vi "Find Type.vi"(8 "error in":errorcluster, 11 "Actor In":refnum<class "Actor.lvclass">) -> (0 "error out":errorcluster, 1 "Type Found?":bool, 2 "Entity Type":T1, 3 "Actor Out":refnum<class "Actor.lvclass">)   [LabVIEW 2020]
doc: "Determines the type of <b>Actor In</b>"
uses:
  <vilib>/ActorFramework/Actor/Actor.lvclass
  Classes/Coffee Shop/Entity Types.ctl
  Classes/Person/Person.lvclass
  Classes/Customer/Customer.lvclass
  Classes/Worker/Worker.lvclass
  Classes/Worker/Barista/Barista.lvclass
  Classes/Worker/Cashier/Cashier.lvclass
  Classes/Coffee Shop/Coffee Shop.lvclass
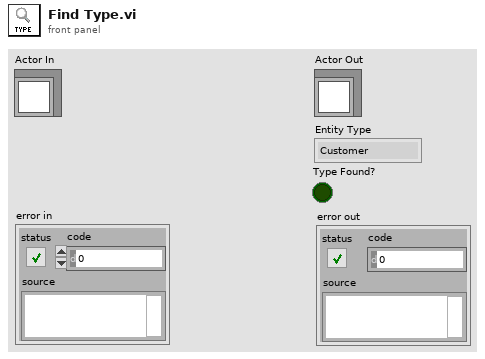
[diagram p1: front panel]
types:
  T1 = typedef "Coffee Shop.lvlib/Coffee Shop.lvclass/Entity Types.ctl" = enum16{"Customer", "Cashier", "Barista"}
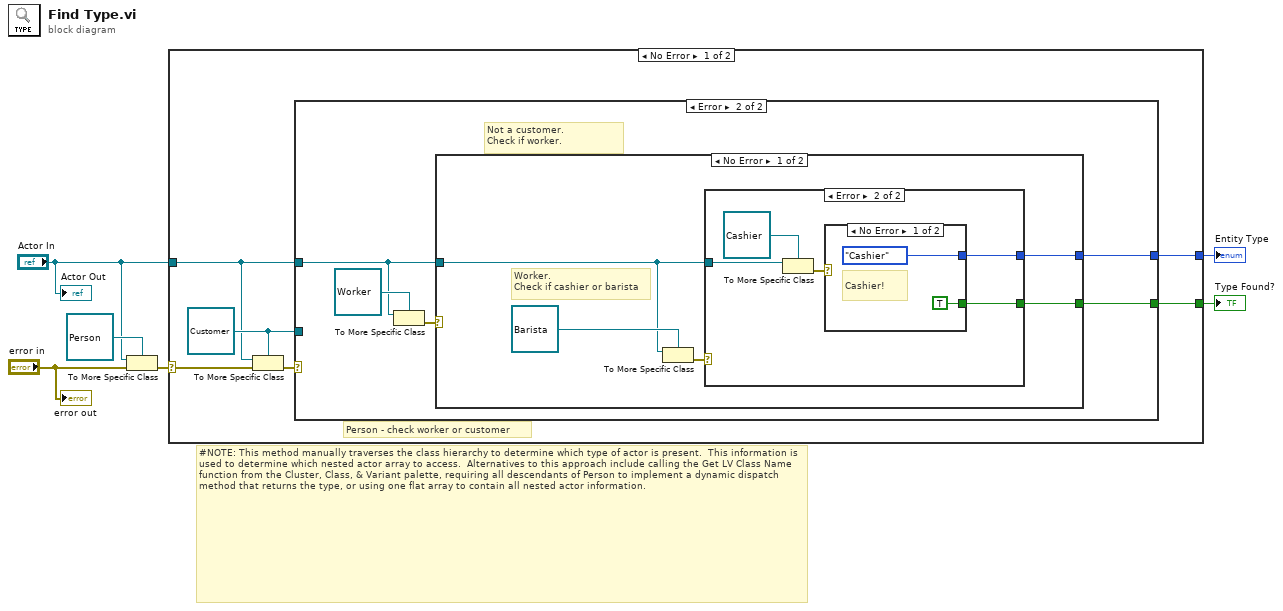
[diagram p0: block diagram]
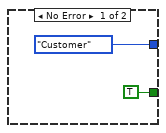
[diagram p2: hidden frame]
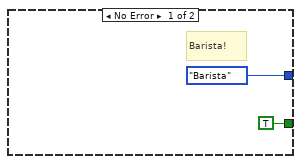
[diagram p3: hidden frame]
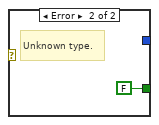
[diagram p4: hidden frame]
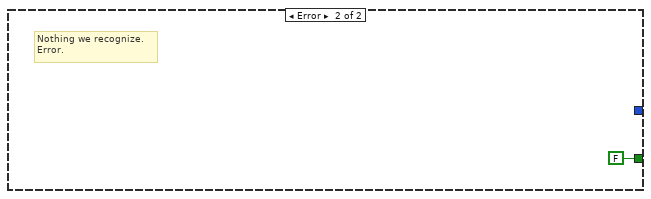
[diagram p5: hidden frame]
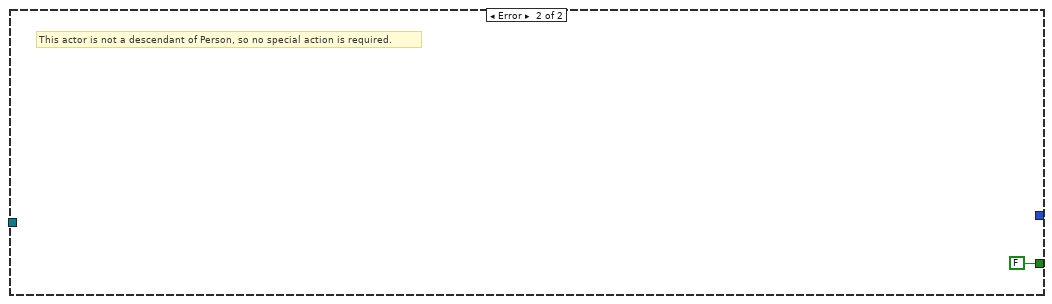
[diagram p6: hidden frame]
diagram:
  # "#NOTE: This method manually traverses the class hierarchy to determine which type of actor is present.  This information is used to determine which nested actor array to access.  Alternatives to this approach include calling the Get LV Class Name function from the Cluster, Class, & Variant palette, requiring all descendants of Person to implement a dynamic dispatch method that returns the type, or using one flat array to contain all nested actor information."
  n1 = To More Specific Class(target class=refnum<class "Person.lvclass"> refnum ("Person.lvclass"), reference="Actor In", error in="error in") -> (error out=w5:errorcluster)  [unwired: 1 out]
  n2 = case shown="No Error" w5 {
    selector: w5 -> [w12 _]
    tunnel: "Actor In" -> [w9 _]
    tunnel: [w8 _] -> w2
    tunnel: [w7 FALSE] -> w3
    frame No Error {
      w10 = refnum<class "Customer.lvclass"> refnum ("Customer.lvlib:Customer.lvclass")
      # "Person - check worker or customer"
      n3 = To More Specific Class(target class=w10, reference=w9, error in=w12) -> (error out=w11:errorcluster)  [unwired: 1 out]
      n4 = case shown="Error" w11 {
        tunnel: w10 -> [_ _]
        tunnel: w9 -> [_ w17]
        tunnel: [Entity_Types."Customer" ("Entity Type") w15] -> w8
        tunnel: [TRUE w16] -> w7
        frame No Error {
        }
        frame Error {
          # "Not a customer.\nCheck if worker."
          n5 = To More Specific Class(target class=refnum<class "Worker.lvclass"> refnum ("Workers.lvlib:Worker.lvclass"), reference=w17) -> (error out=w18:errorcluster)  [unwired: 1 in, 1 out]
          n6 = case shown="No Error" w18 {
            tunnel: w17 -> [w21 _]
            tunnel: [w22 FALSE] -> w16
            tunnel: [w20 _] -> w15
            frame No Error {
              # "Worker.\nCheck if cashier or barista"
              n7 = To More Specific Class(target class=refnum<class "Barista.lvclass"> refnum ("Workers.lvlib:Barista.lvclass"), reference=w21) -> (error out=w23:errorcluster)  [unwired: 1 in, 1 out]
              n8 = case shown="Error" w23 {
                tunnel: [TRUE w27] -> w22
                tunnel: w21 -> [_ w31]
                tunnel: [Entity_Types."Barista" ("Entity Type") w28] -> w20
                frame No Error {
                  # "Barista!"
                }
                frame Error {
                  n9 = To More Specific Class(target class=refnum<class "Cashier.lvclass"> refnum ("Workers.lvlib:Cashier.lvclass"), reference=w31) -> (error out=w29:errorcluster)  [unwired: 1 in, 1 out]
                  n10 = case shown="No Error" w29 {
                    tunnel: [Entity_Types."Cashier" ("Entity Type") _] -> w28
                    tunnel: [TRUE FALSE] -> w27
                    frame No Error {
                      # "Cashier!"
                    }
                    frame Error {
                      # "Unknown type."
                    }
                  }
                }
              }
            }
            frame Error {
              # "Nothing we recognize.\nError."
            }
          }
        }
      }
    }
    frame Error {
      # "This actor is not a descendant of Person, so no special action is required."
    }
  }
  "Type Found?" <- w3
  "Entity Type" <- w2
  "error out" <- "error in"
  "Actor Out" <- "Actor In"
